vi "FTW-TestStep-Base_ReportResults.vi"(0 "FTW-ScripterStep-Base In":refnum<class "FTW-TestStep-Base.lvclass">, 5 "Passed":bool, 7 "Additional Results":variant, 11 "error in (no error)":errorcluster) -> (4 "FTW-ScripterStep-Base Out":refnum<class "FTW-TestStep-Base.lvclass">, 15 "error out":errorcluster)   [LabVIEW 2015, in "FTW-TestStep-Base.lvclass"]
uses:
  FTW-TestStep-Base.lvclass
  Test Executive/FTW-TestExecutive-Results.ctl
  source/container/FTW-Container.lvclass
  FTW-TestStep-Base.lvclass/FTW-TestStep-Base.ctl
  source/actor/Connector/FTW-ActorConnector.lvclass
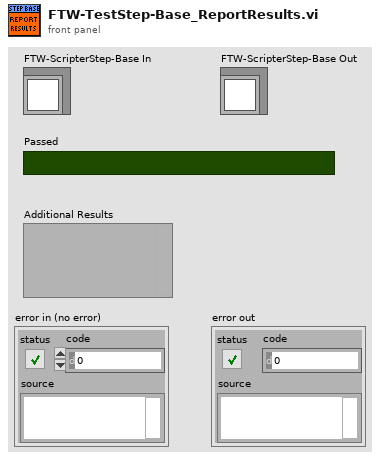
[diagram p1: front panel]
types:
  T1 = typedef "FTW-TestExecutive-Results.ctl" = cluster{"Start Time":timestamp, "Elapsed Time":dbl, "Passed":bool, "Additional Results":refnum<class "FTW-Container.lvclass">}
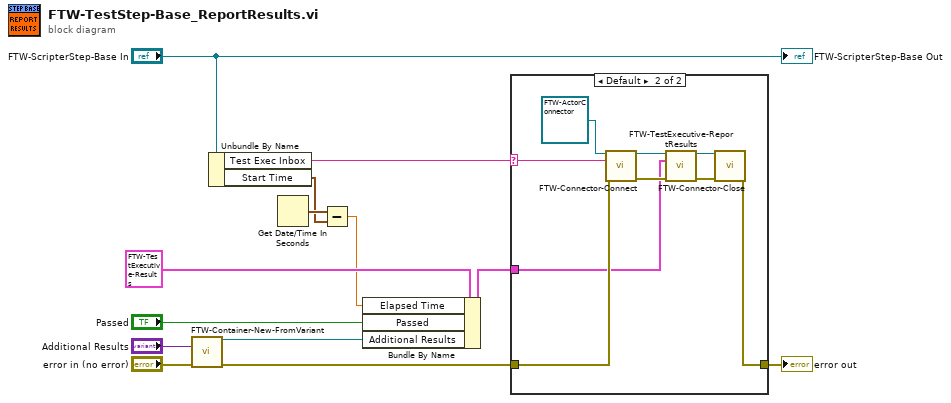
[diagram p0: block diagram]
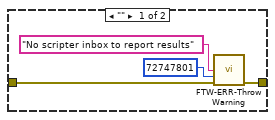
[diagram p2: hidden frame]
diagram:
  n1 = call "FTW-Container-New-FromVariant.vi"("Variant"="Additional Results", "error in"="error in (no error)") -> ("FTW-Container"=w8:refnum<class "FTW-Container.lvclass">, "error out"=w10:errorcluster)  [unwired: 12 in]
  n2 = Unbundle By Name("FTW-ScripterStep-Base In") -> ("Test Exec Inbox"=w4:string, "Start Time"=w2:timestamp)
  n3 = Get Date/Time In Seconds() -> (seconds since 1Jan1904=w3:timestamp)
  n4 = Subtract(x=w3, y=w2) -> (x-y=w1:dbl)
  n5 = Bundle By Name(cluster=T1 {"Start Time"=timestamp(0 s since 1904-01-01), "Elapsed Time"=0.0, "Passed"=FALSE, "Additional Results"=refnum} ("Results"), "Elapsed Time"=w1, "Passed"="Passed", "Additional Results"=w8) -> (w7:T1)
  n6 = case shown="Default" w4 {
    selector: w4 -> [_ w18]
    tunnel: [w16 w23] -> w13
    tunnel: w10 -> [w17 w20]
    tunnel: w7 -> [_ w19]
    frame "" {
      n7 = call "FTW-ERR-ThrowWarning.vi"("Warning Message"="No scripter inbox to report results" ("Error Message"), "Error Code"=72747801, "error in"=w17) -> ("error out"=w16:errorcluster)  [unwired: 12 in]
    }
    frame Default {
      n8 = call-dynamic "FTW-Connector-Connect.vi"("FTW Actor Connector Type"=refnum<class "FTW-ActorConnector.lvclass"> refnum, "Instance Inbox Address"=w18, "error in"=w20) -> ("FTW Actor Connector"=w25:refnum<class "FTW-ActorConnector.lvclass">, "error out"=w21:errorcluster)  [unwired: 11 in]
      n9 = call "FTW-TestExecutive-ReportResults.vi"("FTW Actor Connector In"=w25, "Results"=w19, "error in (no error)"=w21) -> ("FTW Actor Connector"=w26:refnum<class "FTW-ActorConnector.lvclass">, "error out"=w24:errorcluster)  [unwired: 9 in, 2 out]
      n10 = call-dynamic "FTW-Connector-Close.vi"("FTW Actor Connector"=w26, "error in"=w24) -> ("error out"=w23:errorcluster)  [unwired: 13 in]
    }
  }
  "error out" <- w13
  "FTW-ScripterStep-Base Out" <- "FTW-ScripterStep-Base In"
